vi "内置参数对话框.vi"() -> ()   [LabVIEW 2016, in "超标留样集成.lvlib" / "ESTD1200.lvlib"]
uses:
  ESTD1200.lvlib
  <vilib>/Plasmionique/MB Master/MB Master.lvlib
panel:
  in  "退出":bool
  in  "采样器SN号":string
  in  "MODBUS地址":u16
  in  "波特率":u16
  in  "进样超时时间(单位s)":u16
  in  "进样管路排空时间(单位s)":u16
  in  "润洗时间(单位s)":u16
  in  "采样泵速度(默认3500Hz)":u16
  in  "转盘电机偏移补偿量(角度)":i16
  in  "转盘电机速度(默认600Hz)":u16
  in  "电机排液时间(单位s)":u16
  in  "采排液电机速度(默认3000Hz)":u16
  # "内置参数"
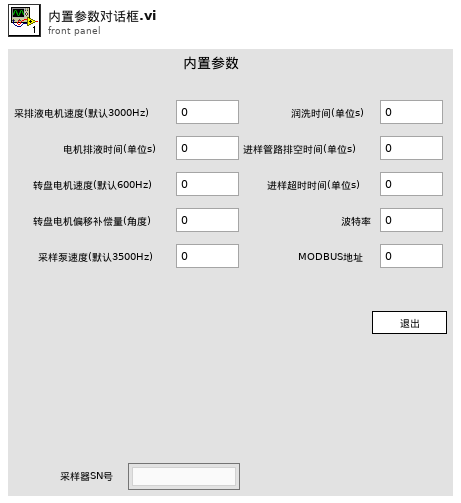
[diagram p1: front panel]
types:
  T1 = cluster{"采排液电机速度":u16, "采排液电机:排液时间":u16, "转盘电机速度":u16, "转盘电机偏移量补偿":i16, "采样泵速度":u16, "润洗时间":u16, "进样管路排空时间":u16, "进样超时时间":u16, "波特率":u16, "MODBUS地址":u16, "校准时间":timestamp, "SN号":string}
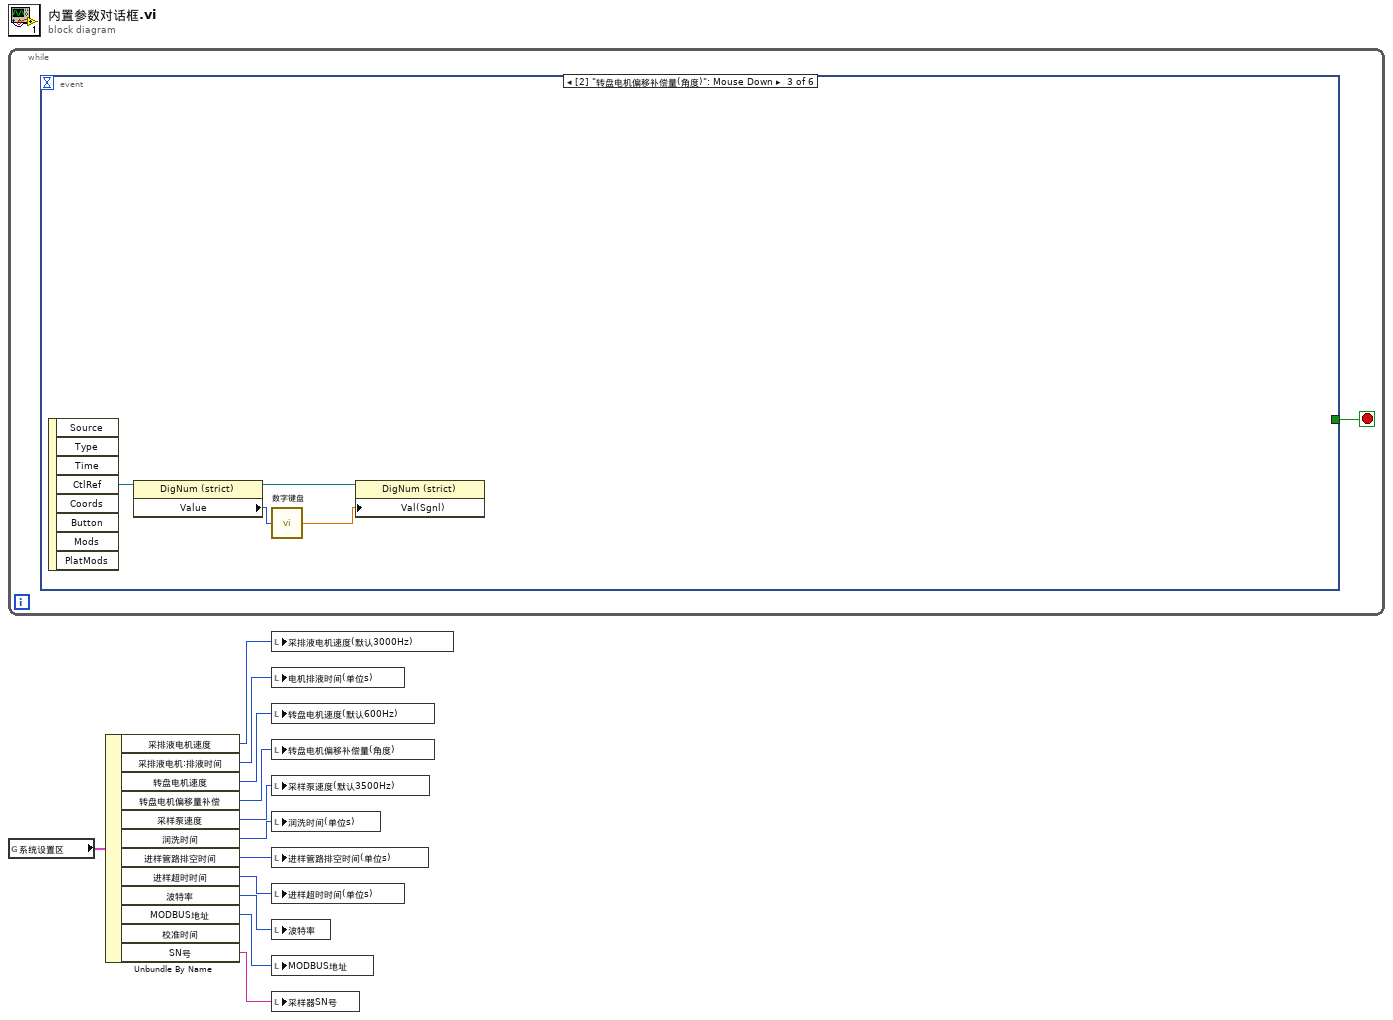
[diagram p0: block diagram]
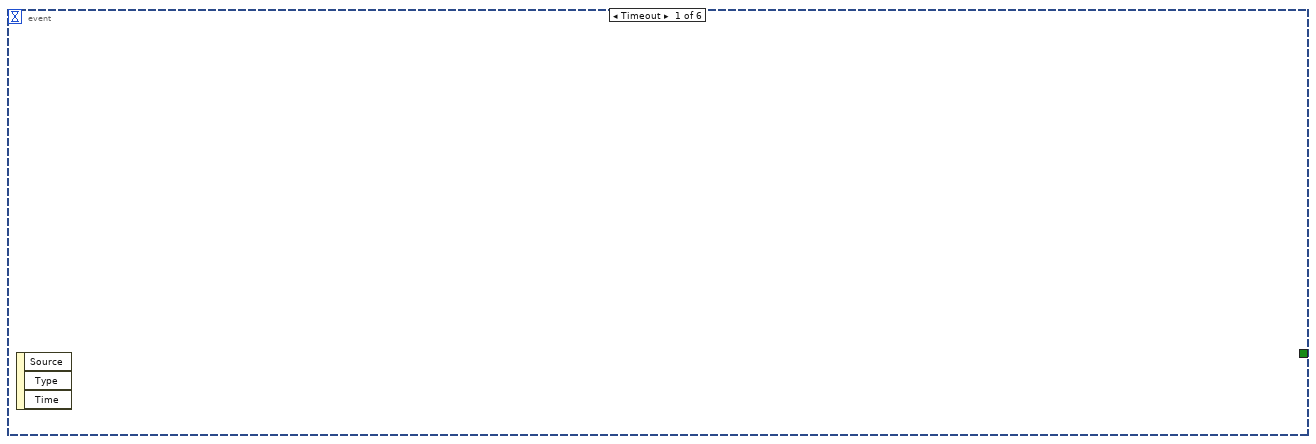
[diagram p2: hidden frame]
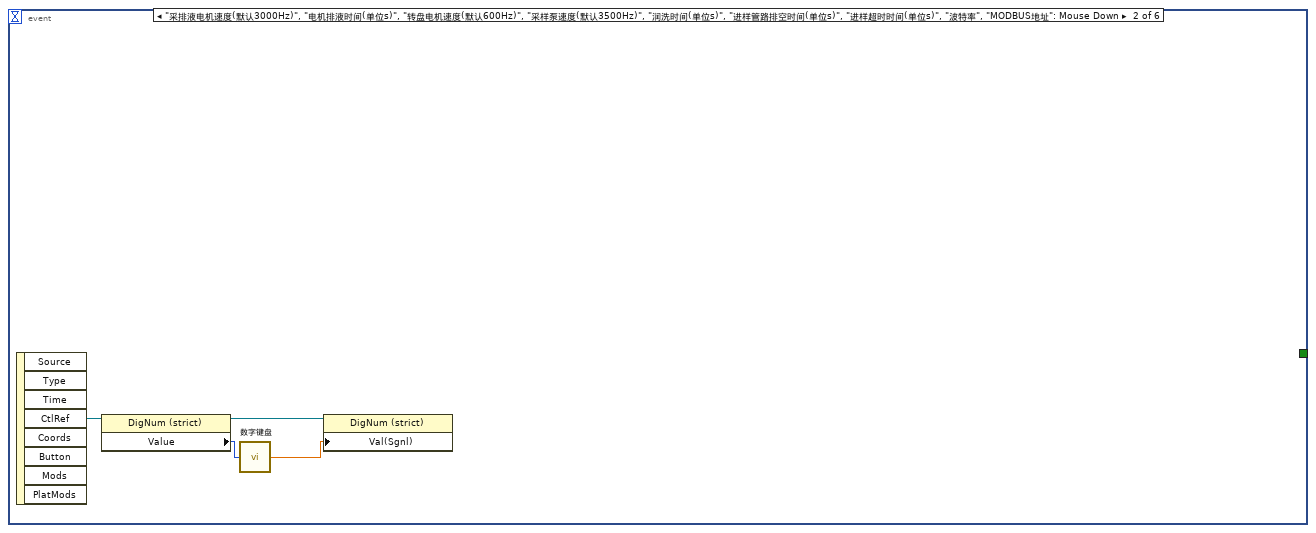
[diagram p3: hidden frame]
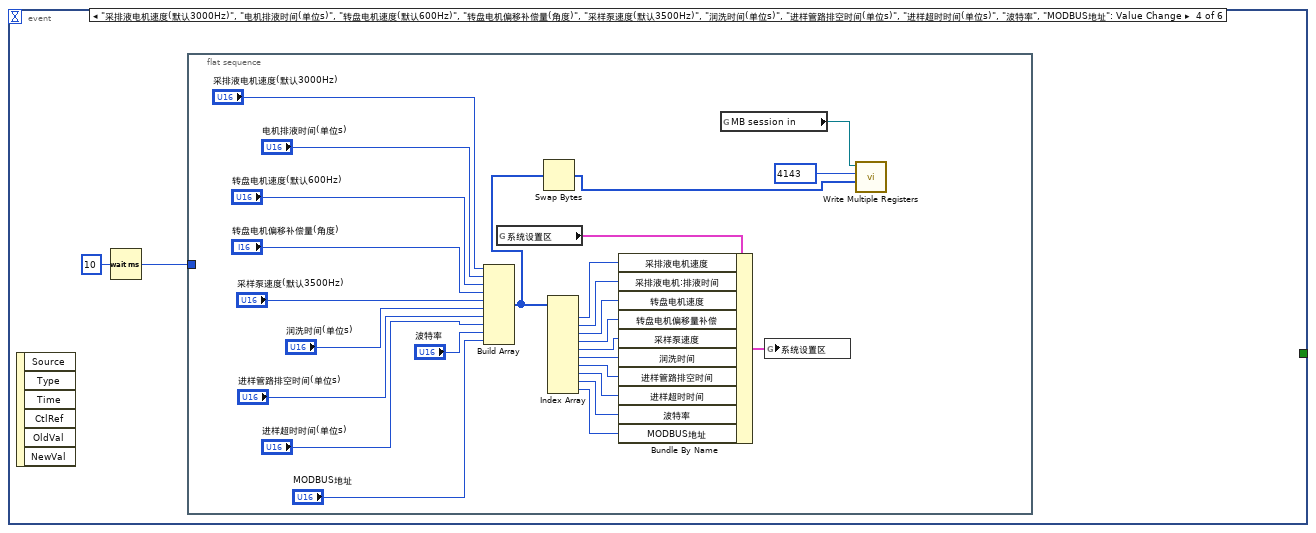
[diagram p4: hidden frame]
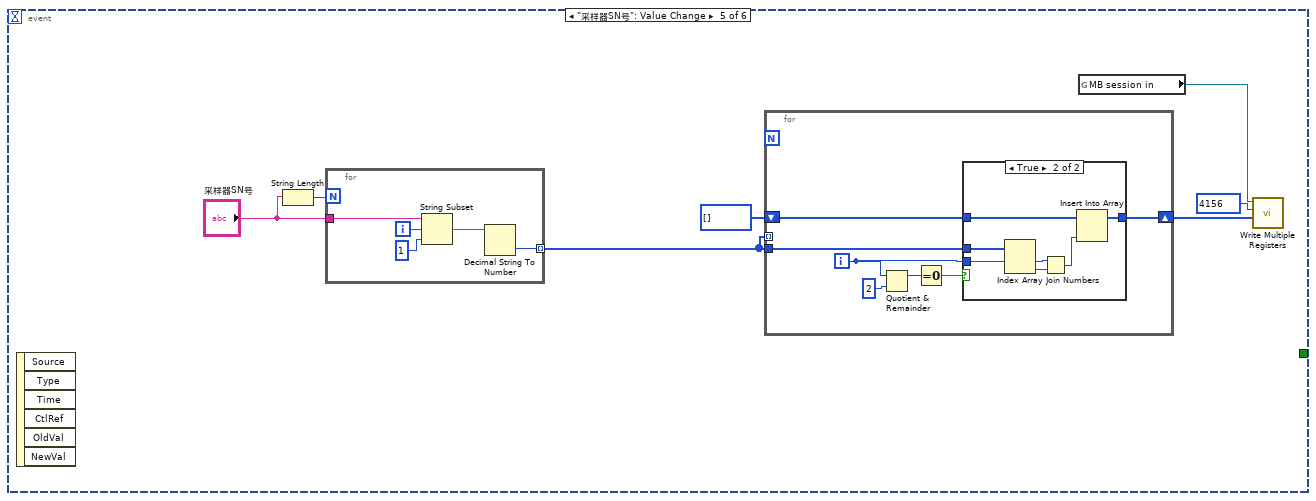
[diagram p5: hidden frame]
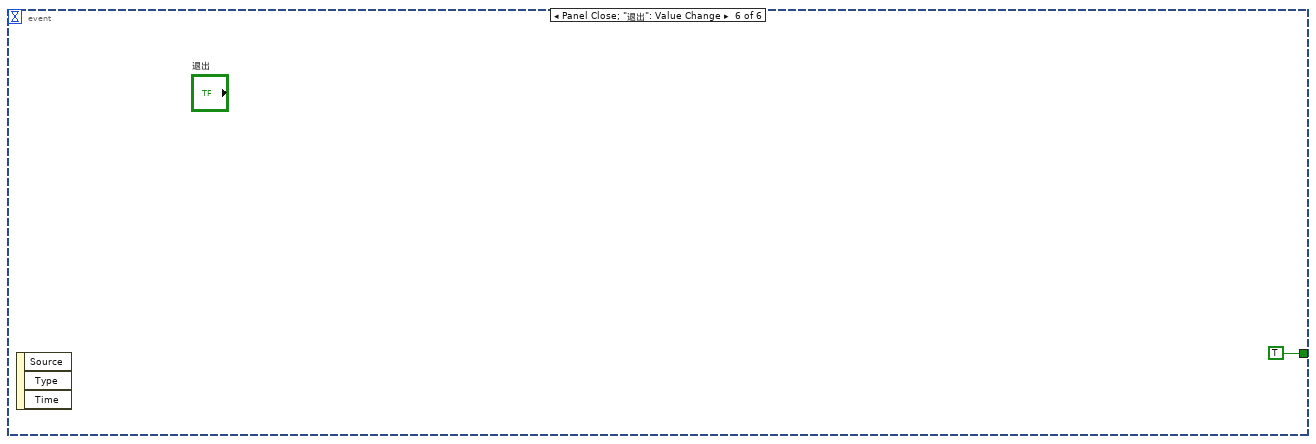
[diagram p7: hidden frame]
diagram:
  n1 = while {
    stop <- w13 stop-if-true
    n2 = event shown="[2] \"转盘电机偏移补偿量(角度)\": Mouse Down" {
      selector: _ -> [_ _ _ _ _ _]
      dyn-events: _ -> [_ _ _ _ _ _]
      timeout: _ -> [_ _ _ _ _ _]
      tunnel: [_ _ _ _ _ TRUE] -> w13
      event Timeout {
        n3 = event-data() -> ()  [unwired: 1 in, 3 out]
      }
      event "采排液电机速度(默认3000Hz)", "电机排液时间(单位s)", "转盘电机速度(默认600Hz)", "采样泵速度(默认3500Hz)", "润洗时间(单位s)", "进样管路排空时间(单位s)", "进样超时时间(单位s)", "波特率", "MODBUS地址": Mouse Down {
        n4 = event-data() -> ("CtlRef"=w17:refnum<vi>)  [unwired: 1 in, 7 out]
        n5 = property class="DigNum (strict)"(reference=w17) -> (reference out=w15:refnum<vi>, "Value"=w16:u16)  [unwired: 1 in, 1 out]
        n6 = call "数字键盘.vi"("OldNumber"=w16) -> ("NewNumber"=w14:sgl)
        n7 = property class="DigNum (strict)"(reference=w15, "Val(Sgnl)"=w14) -> ()  [unwired: 1 in, 2 out]
      }
      event "转盘电机偏移补偿量(角度)": Mouse Down {
        n8 = event-data() -> ("CtlRef"=w21:refnum<vi>)  [unwired: 1 in, 7 out]
        n9 = property class="DigNum (strict)"(reference=w21) -> (reference out=w19:refnum<vi>, "Value"=w20:i16)  [unwired: 1 in, 1 out]
        n10 = call "数字键盘.vi"("OldNumber"=w20) -> ("NewNumber"=w18:sgl)
        n11 = property class="DigNum (strict)"(reference=w19, "Val(Sgnl)"=w18) -> ()  [unwired: 1 in, 2 out]
      }
      event "采排液电机速度(默认3000Hz)", "电机排液时间(单位s)", "转盘电机速度(默认600Hz)", "转盘电机偏移补偿量(角度)", "采样泵速度(默认3500Hz)", "润洗时间(单位s)", "进样管路排空时间(单位s)", "进样超时时间(单位s)", "波特率", "MODBUS地址": Value Change {
        n12 = event-data() -> ()  [unwired: 1 in, 6 out]
        n13 = Wait (ms)(milliseconds to wait=u32 10 ("等待时间（毫秒）")) -> (millisecond timer value=w22:u32)
        n14 = flat-sequence {
          tunnel: w22 -> [_]
          frame #0 {
            n15 = Build Array("采排液电机速度(默认3000Hz)", "电机排液时间(单位s)", "转盘电机速度(默认600Hz)", "转盘电机偏移补偿量(角度)", "采样泵速度(默认3500Hz)", "润洗时间(单位s)", "进样管路排空时间(单位s)", "进样超时时间(单位s)", "波特率", "MODBUS地址") -> (w49:u16[])
            n16 = global read "超标留样全局.vi" "系统设置区"() -> (w38:T1)
            n17 = Swap Bytes(anything=w49) -> (byte swapped=w24:u16[])
            n18 = Index Array(array=w49) -> (element #1=w37:u16, element #2=w36:u16, element #3=w35:u16, element #4=w34:u16, element #5=w33:u16, element #6=w32:u16, element #7=w31:u16, element #8=w30:u16, element #9=w29:u16, element #10=w28:u16)  [unwired: 10 in]
            n19 = Bundle By Name(cluster=w38, "采排液电机速度"=w37, "采排液电机:排液时间"=w36, "转盘电机速度"=w35, "转盘电机偏移量补偿"=w34, "采样泵速度"=w33, "润洗时间"=w32, "进样管路排空时间"=w31, "进样超时时间"=w30, "波特率"=w29, "MODBUS地址"=w28) -> (w27:T1)
            n20 = global read "超标留样全局.vi" "MB session in"() -> (w25:refnum<class "MB_Master.lvclass">)
            n21 = global write "超标留样全局.vi" "系统设置区"(w27) -> ()
            n22 = call <vilib>:"Write Multiple Registers.vi"("values"=w24, "starting address"=u16 4143, "MB session in"=w25) -> ()  [unwired: 7 in, 2 out]
          }
        }
      }
      event "采样器SN号": Value Change {
        n23 = event-data() -> ()  [unwired: 1 in, 6 out]
        n24 = String Length(string="采样器SN号") -> (length=w54:i32)
        n25 = for {
          N: w54 -> [_]
          tunnel: "采样器SN号" -> [w75]
          tunnel: [w72] -> w51 mode=indexing
          i -> [w74]
          n26 = String Subset(string=w75, offset (0)=w74, length (rest)=1 ("长度（剩余）")) -> (substring=w73:string)
          n27 = Decimal String To Number(string=w73) -> (number=w72:i32)  [unwired: 2 in, 1 out]
        }
        n28 = for {
          tunnel: w51 -> [_] mode=indexing
          tunnel: w51 -> [w60]
          shift-right: [w57] -> w50
          shift-left: u16[] [] -> [w58]
          i -> [w59]
          n29 = Quotient & Remainder(x=w59, y=2) -> (x-y*floor(x/y)=w62:i32)  [unwired: 1 out]
          n30 = Equal To 0?(x=w62) -> (x = 0?=w61:bool)
          n31 = case shown="True" w61 {
            tunnel: w60 -> [_ w71]
            tunnel: w59 -> [_ w70]
            tunnel: w58 -> [w64 w67]
            tunnel: [w64 w65] -> w57
            frame False {
            }
            frame True {
              n32 = Index Array(array=w71, index #1=w70) -> (element #1=w69:i32, element #2=w68:i32)  [unwired: 1 in]
              n33 = Join Numbers(hi=w69, lo=w68) -> ((hi.lo)=w66:u64)
              n34 = Insert Into Array(array=w67, new element=w66) -> (w65:u16[])  [unwired: 1 in]
            }
          }
        }
        n35 = global read "超标留样全局.vi" "MB session in"() -> (w55:refnum<class "MB_Master.lvclass">)
        n36 = call <vilib>:"Write Multiple Registers.vi"("values"=w50, "starting address"=u16 4156, "MB session in"=w55) -> ()  [unwired: 7 in, 2 out]
      }
      event Panel Close; "退出": Value Change {
        n37 = event-data() -> ()  [unwired: 1 in, 3 out]
      }
    }
  }
  n38 = global read "超标留样全局.vi" "系统设置区"() -> (w12:T1)
  n39 = Unbundle By Name(w12) -> ("采排液电机速度"=w11:u16, "采排液电机:排液时间"=w10:u16, "转盘电机速度"=w9:u16, "转盘电机偏移量补偿"=w8:i16, "采样泵速度"=w7:u16, "润洗时间"=w6:u16, "进样管路排空时间"=w5:u16, "进样超时时间"=w4:u16, "波特率"=w3:u16, "MODBUS地址"=w2:u16, "SN号"=w1:string)  [unwired: 1 out]
  n40 = local write "采排液电机速度(默认3000Hz)"(w11) -> ()
  n41 = local write "电机排液时间(单位s)"(w10) -> ()
  n42 = local write "转盘电机速度(默认600Hz)"(w9) -> ()
  n43 = local write "转盘电机偏移补偿量(角度)"(w8) -> ()
  n44 = local write "采样泵速度(默认3500Hz)"(w7) -> ()
  n45 = local write "润洗时间(单位s)"(w6) -> ()
  n46 = local write "进样管路排空时间(单位s)"(w5) -> ()
  n47 = local write "进样超时时间(单位s)"(w4) -> ()
  n48 = local write "波特率"(w3) -> ()
  n49 = local write "MODBUS地址"(w2) -> ()
  n50 = local write "采样器SN号"(w1) -> ()
